vi "VP CA LOAD.vi"(0 "path":path) -> (1 "VP Output Names":string[](array[string]), 2 "CA Output Numbers":i32[](array[numeric]), 3 "CA Input Numbers":i32[](array[numeric]), 4 "VALID":bool, 5 "VP Input Names":string[](array[string]), 6 "CA Output Names":string[](array[string]), 7 "CA Input Names":string[](array[string]))   [LabVIEW 2019]
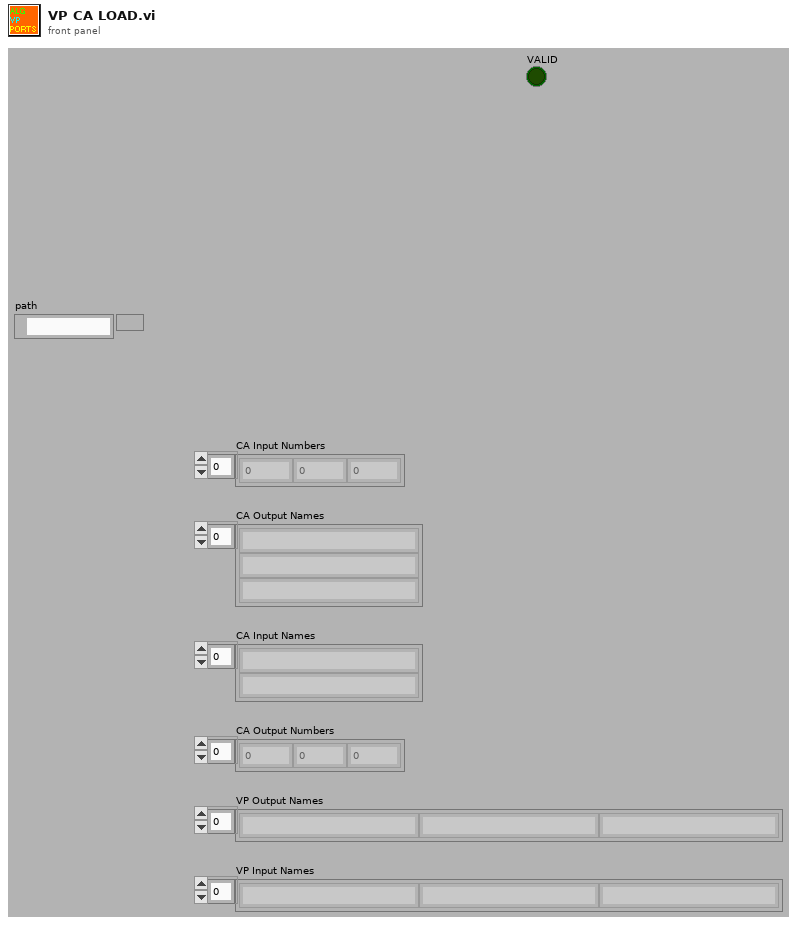
[diagram p1: front panel]
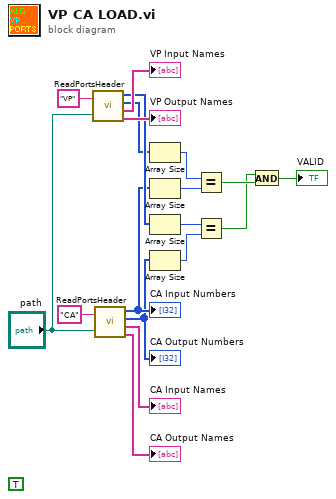
[diagram p0: block diagram]
diagram:
  (unwired) TRUE
  n1 = call "ReadPortsHeader.vi"("base path"="path", "FileName"="VP" ("name or relative path")) -> ("Output Names"=→"VP Output Names":string[], "Input Names"=→"VP Input Names":string[], "Output Numbers"=w6:i32[], "Input Numbers"=w11:i32[])
  n2 = call "ReadPortsHeader.vi"("base path"="path", "FileName"="CA" ("name or relative path")) -> ("Output Names"=→"CA Output Names":string[], "Input Names"=→"CA Input Names":string[], "Output Numbers"=w2:i32[], "Input Numbers"=w3:i32[])
  "CA Input Numbers" <- w3
  "CA Output Numbers" <- w2
  n3 = Array Size(array=w6) -> (size(s)=w7:i32)
  n4 = Array Size(array=w3) -> (size(s)=w8:i32)
  n5 = Array Size(array=w11) -> (size(s)=w10:i32)
  n6 = Array Size(array=w2) -> (size(s)=w9:i32)
  n7 = Equal?(x=w7, y=w8) -> (x = y?=w5:bool)
  n8 = Equal?(x=w10, y=w9) -> (x = y?=w4:bool)
  n9 = And(x=w4, y=w5) -> (x .and. y?=→"VALID":bool)
